vi "PCT Configure Enqueue CMD.vi"(5 "Response Queue":refnum<queue>, 6 "Parameter Data":variant, 7 "Read":bool, 8 "error in (no error)":errorcluster, 9 "Priority Message? (F)":bool, 10 "CMD":T1={"Type CMD"="Trace", "Mode CMD"="Swept SA", "Main CMD"="Data"}, 11 "CMD Queue in":refnum<queue>) -> (0 "error out":errorcluster, 3 "CMD Queue out":refnum<queue>, 4 "Message Data":variant)   [LabVIEW 2020, in "Message Queue.lvlib"]
uses:
  Message Queue/Message Queue.lvlib
  Message Queue/Message Cluster.ctl
  HW Message Cluster.ctl
  Message Queue/Enqueue Message (Single).vi
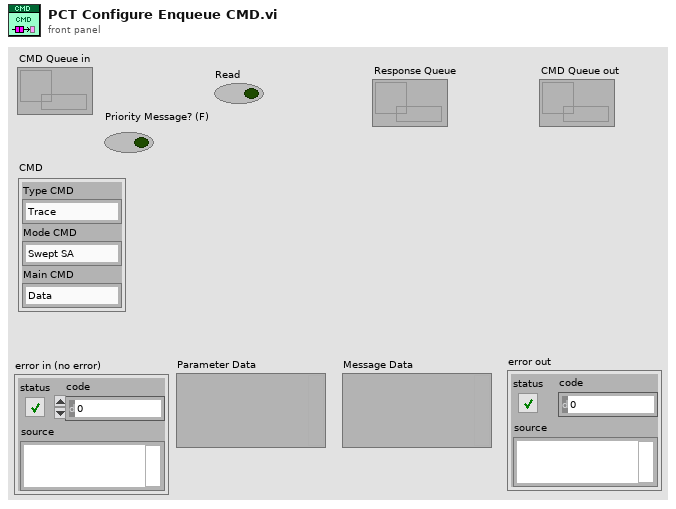
[diagram p1: front panel]
types:
  T1 = cluster{"Type CMD":string, "Mode CMD":string, "Main CMD":string}
  T2 = typedef "Message Queue.lvlib/HW Message Cluster.ctl" = cluster{"Writer Queue":refnum<queue>, "Writer Data":T3}
  T3 = typedef "Message Queue.lvlib/Message Cluster.ctl" = cluster{"Message":string, "Message Data":variant}
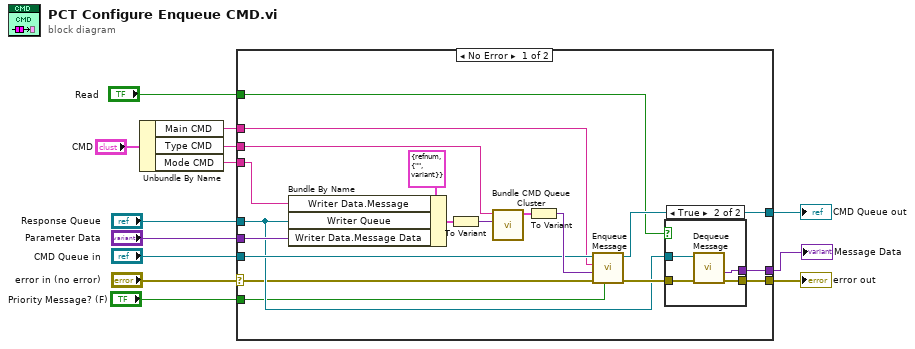
[diagram p0: block diagram]
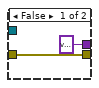
[diagram p2: hidden frame]
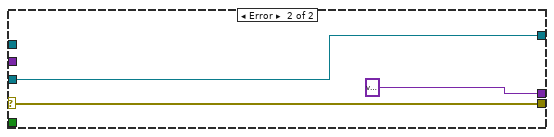
[diagram p3: hidden frame]
diagram:
  n1 = Unbundle By Name("CMD") -> ("Main CMD"=w5:string, "Type CMD"=w6:string, "Mode CMD"=w4:string)
  n2 = case shown="No Error" "error in (no error)" {
    selector: "error in (no error)" -> [w19 w40]
    tunnel: "Response Queue" -> [w20 _]
    tunnel: [w31 w39] -> w12
    tunnel: [w22 w40] -> w11
    tunnel: "CMD Queue in" -> [w29 w39]
    tunnel: w6 -> [w18 _]
    tunnel: w4 -> [w25 _]
    tunnel: "Parameter Data" -> [w27 _]
    tunnel: w5 -> [w26 _]
    tunnel: "Read" -> [w24 _]
    tunnel: [w21 variant ("Message Data")] -> w3
    tunnel: "Priority Message? (F)" -> [w14 _]
    frame No Error {
      n3 = Bundle By Name(cluster=T2 {"Writer Queue"=refnum, "Writer Data"={"Message"="", "Message Data"=variant}} ("HW Message"), "Writer Data.Message"=w25, "Writer Queue"=w20, "Writer Data.Message Data"=w27) -> (w28:T2)
      n4 = To Variant(anything=w28) -> (Variant=w17:variant)
      n5 = call "Bundle CMD Queue Cluster.vi"("Message Data"=w17, "Message"=w18) -> ("Message Cluster"=w16:T3)  [unwired: 9 in]
      n6 = To Variant(anything=w16) -> (Variant=w30:variant)
      n7 = call-poly "Enqueue Message.vi"("Priority Message? (F)"=w14, "error in (no error)"=w19, "Message Data"=w30, "Message"=w26, "Message Queue"=w29) -> ("error out"=w23:errorcluster, "dup Message Queue"=w31:refnum<queue>)  [unwired: 5 in]
      n8 = case shown="True" w24 {
        tunnel: w20 -> [_ w37]
        tunnel: w23 -> [w33 w36]
        tunnel: [w33 w35] -> w22
        tunnel: [variant ("Message Data") w34] -> w21
        frame False {
        }
        frame True {
          n9 = call "Dequeue Message.vi"("error in (no error)"=w36, "Message Queue"=w37) -> ("error out"=w35:errorcluster, "Message Data"=w34:variant)  [unwired: 6 in, 2 out]
        }
      }
    }
    frame Error {
    }
  }
  "CMD Queue out" <- w12
  "error out" <- w11
  "Message Data" <- w3
